vi "Close.vi"(8 "error in (no error)":errorcluster, 11 "VISA resource name":refnum<visa-resource-name>) -> (0 "error out":errorcluster)   [LabVIEW 2015, in "ZhiYuan ZDS Series for TCP.lvlib"]
doc: "Performs an instrument error query before terminating the software connection to the instrument."
uses:
  ZhiYuan ZDS Series for TCP.lvlib
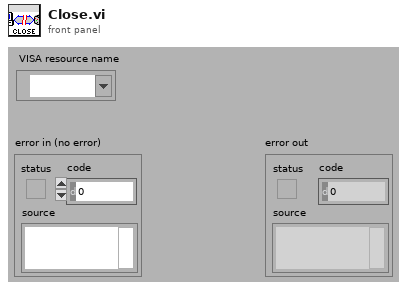
[diagram p1: front panel]
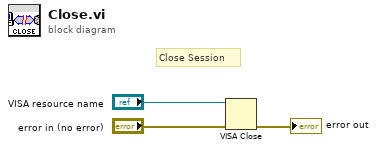
[diagram p0: block diagram]
diagram:
  # "Close Session"
  n1 = VISA Close(VISA resource name="VISA resource name", error in (no error)="error in (no error)") -> (error out=→"error out":errorcluster)
